vi "configureAcquisition.vi"(6 "imagePaths":path[](array[path]), 7 "saveImages?":bool, 8 "error in (no error)":errorcluster, 9 "number of Images":i32, 10 "CameraSettings":refnum<class "CamaraSettings.lvclass">, 11 "ProEM_WinX32 in":refnum<class "ProEM_WinX32.lvclass">) -> (0 "error out":errorcluster, 3 "ProEM_WinX32 out":refnum<class "ProEM_WinX32.lvclass">)   [LabVIEW 2011, in "Hardware.lvlib" / "Channels.lvlib" / "ProEM_WinX32.lvclass"]
doc: "Camera Settings are made from within WinX32 software.\nThey are not changed here.\nOnly the total number of images to take in the acquisition is set from here"
uses:
  ProEM_WinX32.lvclass
  Tools/CameraSettings/CamaraSettings.lvclass
  ProEM_WinX32.lvclass/ProEM_WinX32.ctl
  Camera/Camera.lvclass
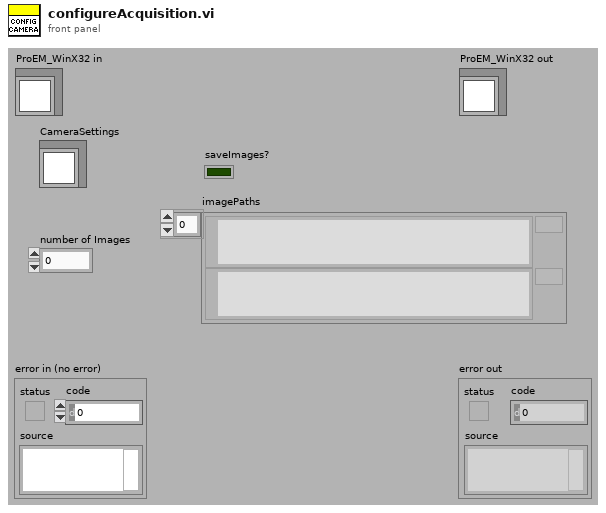
[diagram p1: front panel]
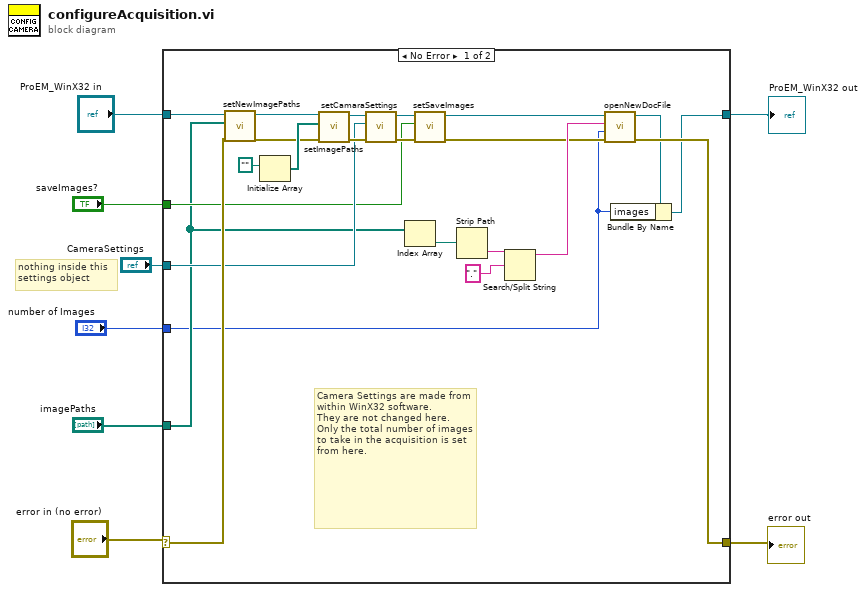
[diagram p0: block diagram]
diagram:
  # "nothing inside this\nsettings object"
  n1 = case shown="No Error" "error in (no error)" {
    selector: "error in (no error)" -> [w30 w32]
    tunnel: [w9 w33] -> w8
    tunnel: "ProEM_WinX32 in" -> [w31 w33]
    tunnel: [w14 w32] -> w5
    tunnel: "saveImages?" -> [w20 _]
    tunnel: "CameraSettings" -> [w23 _]
    tunnel: "number of Images" -> [w11 _]
    tunnel: "imagePaths" -> [w19 _]
    frame No Error {
      # "Camera Settings are made from within WinX32 software.\nThey are not changed here.\nOnly the total number of images to take in the acquisition is set from here."
      n2 = call "setNewImagePaths.vi"("error in (no error)"=w30, "NewImagePaths"=w19, "Camera in"=w31) -> ("error out"=w27:errorcluster, "Camera out"=w26:refnum<class "ProEM_WinX32.lvclass">)  [unwired: 7 in]
      n3 = Initialize Array(path "") -> (w28:path[])  [unwired: 1 in]
      n4 = call "setImagePaths.vi"("error in (no error)"=w27, "ImagePaths"=w28, "Camera in"=w26) -> ("error out"=w24:errorcluster, "Camera out"=w25:refnum<class "ProEM_WinX32.lvclass">)  [unwired: 7 in]
      n5 = call "setCamaraSettings.vi"("error in (no error)"=w24, "CamaraSettings"=w23, "Camera in"=w25) -> ("error out"=w21:errorcluster, "Camera out"=w22:refnum<class "ProEM_WinX32.lvclass">)  [unwired: 7 in]
      n6 = Index Array(array=w19) -> (element=w18:path)  [unwired: 1 in]
      n7 = call "setSaveImages.vi"("error in (no error)"=w21, "saveImages?"=w20, "Camera in"=w22) -> ("error out"=w12:errorcluster, "Camera out"=w13:refnum<class "ProEM_WinX32.lvclass">)  [unwired: 7 in]
      n8 = Strip Path(path=w18) -> (name=w17:string)  [unwired: 1 out]
      n9 = Search/Split String(string=w17, search string/char (-)=".") -> (substring before match=w15:string)  [unwired: 1 in, 2 out]
      n10 = call "openNewDocFile.vi"("error in (no error)"=w12, "# of images"=w11, "name"=w15, "ProEM_WinX32 in"=w13) -> ("error out"=w14:errorcluster, "ProEM_WinX32 out"=w10:refnum<class "ProEM_WinX32.lvclass">)  [unwired: 6 in]
      n11 = Bundle By Name(cluster=w10, "images"=w11) -> (w9:refnum<class "ProEM_WinX32.lvclass">)
    }
    frame Error {
    }
  }
  "error out" <- w5
  "ProEM_WinX32 out" <- w8
